vi "题目3温度测量VI.vi"() -> ()   [LabVIEW 2017]
panel:
  out "温度计":dbl(slide) scale=0.0..200.0
  in  "温度单位":bool
  in  "停止":bool
  in  "温度":string
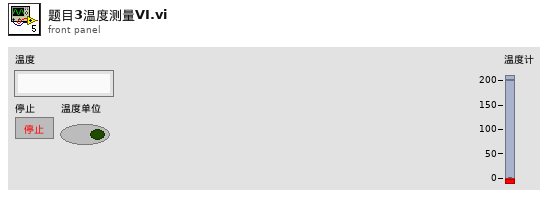
[diagram p1: front panel]
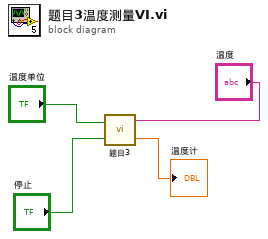
[diagram p0: block diagram]
diagram:
  n1 = call "题目3.vi"("温度"="温度", "停止"="停止", "温度单位"="温度单位") -> ("温度计"=→"温度计":dbl)
